vi "VS-Acquire EKG Sample.vi"(0 "Settings":T1, 7 "Sampling Rate (Hz)":dbl=10000.0) -> (4 "Waveform":dbl[](graph), 15 "error out":errorcluster)   [LabVIEW 2020]
uses:
  Typedefs/PhysMon-HR From EKG Settings.ctl
  epl-vi-lib/Connection VIs/Type Defs/Input sources.ctl
  <vilib>/DAQmx/read.llb/DAQmx Read (Analog 1D DBL 1Chan NSamp).vi
  <vilib>/DAQmx/create/channels.llb/DAQmx Create Channel (AI-Voltage-Basic).vi
  <vilib>/DAQmx/configure/timing.llb/DAQmx Timing (Sample Clock).vi
  <vilib>/DAQmx/miscellaneous.llb/DAQmx Fill In Error Info.vi
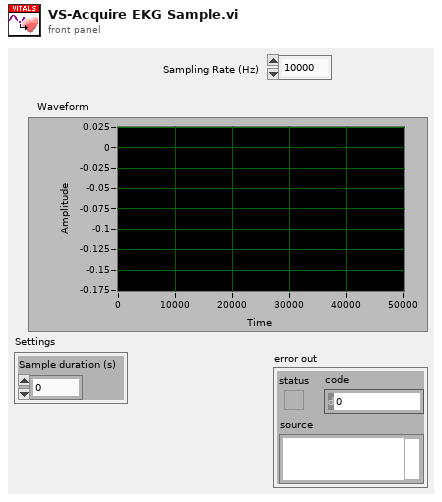
[diagram p1: front panel]
types:
  T1 = typedef "PhysMon-HR From EKG Settings.ctl" = cluster{"Sample duration (s)":dbl}
  T2 = typedef "Input sources.ctl" = u16
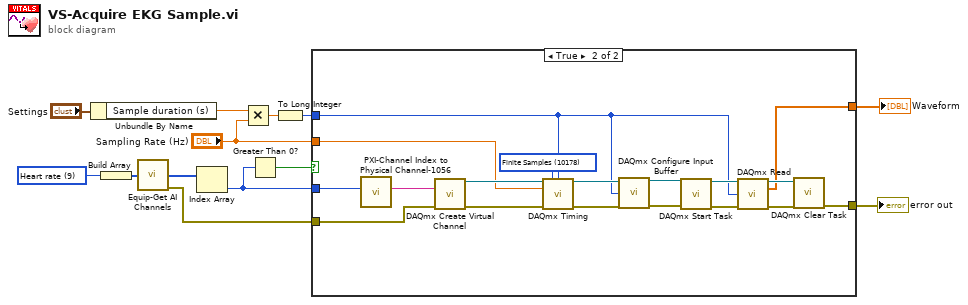
[diagram p0: block diagram]
diagram:
  w8 = T2 9 items=["--unused--", "Probe Mic Right", "Probe Mic Left", "Cal Mic", "ABR", "CAP Right", "CAP Left", "Startle piezo", "Temperature", "Heart rate"] ("Ring")
  n1 = Unbundle By Name("Settings") -> ("Sample duration (s)"=w4:dbl)
  n2 = Build Array(w8) -> (w7:T2[])
  n3 = call "Equip-Get AI Channels.vi"("Inputs"=w7) -> ("AI Channels"=w13:i32[], "error out"=w12:errorcluster)  [unwired: 13 in]
  n4 = Index Array(array=w13) -> (element=w11:i32)  [unwired: 1 in]
  n5 = Multiply(x=w4, y="Sampling Rate (Hz)") -> (x*y=w5:dbl)
  n6 = Greater Than 0?(x=w11) -> (x > 0?=w10:bool)
  n7 = To Long Integer(number=w5) -> (32bit integer=w2:i32)
  n8 = case shown="True" w10 {
    tunnel: w11 -> [_ w18]
    tunnel: [w14 w17] -> w9
    tunnel: w12 -> [w14 w20]
    tunnel: "Sampling Rate (Hz)" -> [_ w16]
    tunnel: w2 -> [_ w19]
    tunnel: [_ w15] -> w1
    frame False {
    }
    frame True {
      w32 = 10178 items=["Finite Samples"=10178, "Continuous Samples"=10123, "Hardware Timed Single Point"=12522] ("sample mode")
      n9 = call "PXI-Channel Index to Physical Channel-1056.vi"("index"=w18) -> ("element"=w21:tag)  [unwired: 10 in]
      n10 = call-poly <vilib>:"DAQmx Create Virtual Channel.vi"("physical channels"=w21, "error in"=w20) -> ("task out"=w26:refnum<k21>, "error out"=w27:errorcluster)  [unwired: 12 in]
      n11 = call-poly <vilib>:"DAQmx Timing.vi"("task/channels in"=w26, "sample mode"=w32, "samples per channel"=w19, "rate"=w16, "error in"=w27) -> ("task out"=w23:refnum<k21>, "error out"=w25:errorcluster)  [unwired: 9 in]
      n12 = call <vilib>:"DAQmx Configure Input Buffer.vi"("task/channels in"=w23, "buffer size (in samples per channel)"=w19, "error in"=w25) -> ("task out"=w22:refnum<k21>, "error out"=w24:errorcluster)  [unwired: 11 in]
      n13 = call <vilib>:"DAQmx Start Task.vi"("task/channels in"=w22, "error in"=w24) -> ("task out"=w28:refnum<k21>, "error out"=w29:errorcluster)  [unwired: 12 in]
      n14 = call-poly <vilib>:"DAQmx Read.vi"("task/channels in"=w28, "number of samples per channel"=w19, "error in"=w29) -> ("task out"=w30:refnum<k21>, "data"=w15:dbl[], "error out"=w31:errorcluster)  [unwired: 10 in]
      n15 = call <vilib>:"DAQmx Clear Task.vi"("task in"=w30, "error in"=w31) -> ("error out"=w17:errorcluster)  [unwired: 13 in]
    }
  }
  "error out" <- w9
  "Waveform" <- w1
